vi "Open Encoders.vi"   [LabVIEW 2019]
uses:
  <vilib>/Rock Robotics/SystemInterfaces/DIO/FPGA_DIOChannel.ctl
  <vilib>/Rock Robotics/WPI/Counter/WPI_CounterDigitalInputToDigitalSource.vi
  <vilib>/Rock Robotics/WPI/Counter/WPI_CounterOpen UpDown Mode.vi
types:
  T1 = typedef "FPGA_DIOChannel.ctl" = enum8{"DIO 0", "DIO 1", "DIO 2", "DIO 3", "DIO 4", "DIO 5", "DIO 6", "DIO 7", "DIO 8", "DIO 9", "DIO MXP 0", "DIO MXP 1", "DIO MXP 2", "DIO MXP 3", "DIO MXP 4", "DIO MXP 5", "DIO MXP 6", "DIO MXP 7", "DIO MXP 8", "DIO MXP 9", "DIO MXP 10", "DIO MXP 11", "DIO MXP 12", "DIO MXP 13", "DIO MXP 14", "DIO MXP 15", "SPI Port CS1", "SPI Port CS2", "SPI Port CS3", "SPI Port MISO", "SPI Port MOSI", "Invalid"}
  T2 = typedef "WPI_DigitalInputDevRef.ctl" = cluster{"DevStatus":errorcluster, "DIO Channel":T1}
  T3 = typedef "FPGA_CounterEncoderSourceConvertionLVSourceType.ctl" = cluster{"DevStatus":errorcluster, "AnalogTriggerMode?":bool, "DigitalMode":cluster{"DIO Channel":T4}, "AnalogTriggerMode":cluster{"AnalogTriggerIndex":T5, "OutputType":T6}}
  T4 = typedef "FPGA_DIODigitalSourceChannel.ctl" = enum8{"DIO 0", "DIO 1", "DIO 2", "DIO 3", "DIO 4", "DIO 5", "DIO 6", "DIO 7", "DIO 8", "DIO 9", "DIO MXP 0", "DIO MXP 1", "DIO MXP 2", "DIO MXP 3", "DIO MXP 4", "DIO MXP 5", "DIO MXP 6", "DIO MXP 7", "DIO MXP 8", "DIO MXP 9", "DIO MXP 10", "DIO MXP 11", "DIO MXP 12", "DIO MXP 13", "DIO MXP 14", "DIO MXP 15", "SPI Port CS1", "SPI Port CS2", "SPI Port CS3", "SPI Port MISO", "SPI Port MOSI", "Disabled"}
  T5 = typedef "FPGA_AnalogTriggerIndex.ctl" = enum8{"Trig 0", "Trig 1", "Trig 2", "Trig 3", "Trig 4", "Trig 5", "Trig 6", "Trig 7", "Invalid"}
  T6 = typedef "FPGA_AnalogTriggerOutType.ctl" = enum16{"InWindow", "TriggerState", "Rising", "Falling"}
  T7 = typedef "WPI_EncoderDevRef.ctl" = cluster{"DevStatus":errorcluster, "EncoderIndex":T8, "CounterIndex":T9, "DistancePerCount":dbl, "Decoding Type":T10}
  T8 = typedef "FPGA_EncoderIdx.ctl" = enum8{"Enc 0", "Enc 1", "Enc 2", "Enc 3", "Enc 4", "Enc 5", "Enc 6", "Enc 7", "Invalid"}
  T9 = typedef "FPGA_CounterCtrSystemIndex.ctl" = enum8{"Ctr 0", "Ctr 1", "Ctr 2", "Ctr 3", "Ctr 4", "Ctr 5", "Ctr 6", "Ctr 7", "Invalid"}
  T10 = typedef "WPI_EncoderType.ctl" = enum16{"1x", "2x", "4x"}
  T11 = typedef "WPI_CounterDevRef.ctl" = cluster{"DevStatus":errorcluster, "CntIndex":T9}
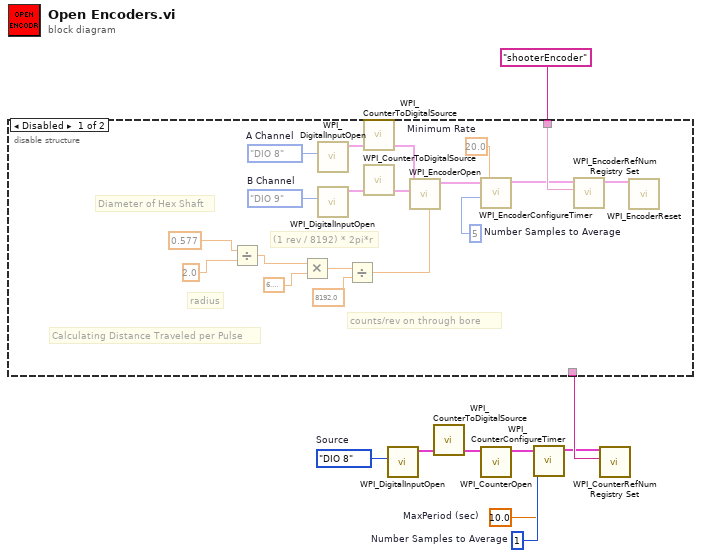
[diagram p0: block diagram]
diagram:
  w1 = 10.0  # MaxPeriod (sec)
  w2 = u8 1  # Number Samples to Average
  w7 = FPGA_DIOChannel."DIO 8"  # Source
  n1 = disable-structure shown="Disabled" {
    disable-tunnel: "shooterEncoder" ("refnum name") -> [w22 w29]
    disable-tunnel: [_ w29] -> w5
    frame Disabled {
      w10 = 20.0  # Minimum Rate
      w18 = u8 5  # Number Samples to Average
      w23 = FPGA_DIOChannel."DIO 9"  # B Channel
      w24 = FPGA_DIOChannel."DIO 8"  # A Channel
      # "(1 rev / 8192) * 2pi*r"
      # "Calculating Distance Traveled per Pulse"
      # "counts/rev on through bore"
      # "radius"
      # "Diameter of Hex Shaft"
      n2 = Divide(x=0.577, y=2.0) -> (x/y=w14:dbl)
      n3 = Multiply(x=w14, y=6.283185307179586) -> (x*y=w13:dbl)
      n4 = call <vilib>:"WPI_DigitalInputOpen.vi"("DIO Channel"=w24) -> ("DigitalInputDevRef"=w27:T2)  [unwired: 1 in, 9 out]
      n5 = call <vilib>:"WPI_DigitalInputOpen.vi"("DIO Channel"=w23) -> ("DigitalInputDevRef"=w26:T2)  [unwired: 1 in, 9 out]
      n6 = Divide(x=w13, y=8192.0) -> (x/y=w11:dbl)
      n7 = call-poly <vilib>:"WPI_CounterToDigitalSource.vi"("DigitalInputDevRef"=w27) -> ("Digital Source"=w28:T3)  [unwired: 6 out]
      n8 = call-poly <vilib>:"WPI_CounterToDigitalSource.vi"("DigitalInputDevRef"=w26) -> ("Digital Source"=w25:T3)  [unwired: 6 out]
      n9 = call <vilib>:"WPI_EncoderOpen.vi"("DistancePerCount"=w11, "BSource"=w25, "ASource"=w28) -> ("EncoderDevRef"=w20:T7)  [unwired: 5 in, 3 out]
      n10 = call <vilib>:"WPI_EncoderConfigureTimer.vi"("Number Samples to Average"=w18, "Minimum Rate"=w10, "EncoderDevRef"=w20) -> ("EncoderDevRef"=w19:T7)  [unwired: 7 in, 1 out]
      n11 = call <vilib>:"WPI_EncoderRefNum Registry Set.vi"("refnum name"=w22, "EncoderDevRef"=w19) -> ("EncoderDevRef"=w21:T7)  [unwired: 8 in, 1 out]
      n12 = call <vilib>:"WPI_EncoderReset.vi"("EncoderDevRef"=w21) -> ()  [unwired: 9 in, 2 out]
    }
    frame Enabled {
    }
  }
  n13 = call <vilib>:"WPI_DigitalInputOpen.vi"("DIO Channel"=w7) -> ("DigitalInputDevRef"=w6:T2)  [unwired: 1 in, 9 out]
  n14 = call-poly <vilib>:"WPI_CounterToDigitalSource.vi"("DigitalInputDevRef"=w6) -> ("Digital Source"=w8:T3)  [unwired: 6 out]
  n15 = call-poly <vilib>:"WPI_CounterOpen.vi"("Up Source"=w8) -> ("CounterDevRef"=w4:T11)  [unwired: 6 in, 4 out]
  n16 = call <vilib>:"WPI_CounterConfigureTimer.vi"("Number Samples to Average"=w2, "MaxPeriod (sec)"=w1, "CounterDevRef in"=w4) -> ("CounterDevRef out"=w3:T11)  [unwired: 7 in, 1 out]
  n17 = call <vilib>:"WPI_CounterRefNum Registry Set.vi"("refnum name"=w5, "CounterDevRef"=w3) -> ()  [unwired: 8 in, 2 out]
